vi "MGI Open Window.vi"(8 "error in (no error)":errorcluster, 9 "Center on Caller? (T)":bool=TRUE, 10 "VI To Center On (Caller)":refnum<vi>, 11 "Behavior (Modal)":T1(ring)=enum."Modal") -> (0 "error out":errorcluster, 3 "Open Initially?":bool)   [LabVIEW 2016]
doc: "Sets the caller VI's behavior as specified (modal as default) and opens its front panel. (Useful so you can keep the VI as non-modal most of the time and thus you will not have problems getting stuck with it open).\n\nBy default, centers the opened VI in it's caller VI (if it's open) but that can be changed using the VI To Center On and Center on Caller? inputs.\n\nAuthor: Hope Harrison\nsupport@mooregoodideas.com\nwww.mooregoodideas.com\n\nCopyright (c) 2016, Moore Good Ideas, Inc.\n\nAll rights reserved.\n\nRedistribution and use in source and binary forms, with or without modification, are permitted provided that the following conditions are met:\n\n * Redistributions of source code must retain the above copyright notice, this list of conditions and the following disclaimer.\n * Redistributions in binary form must reproduce the above copyright notice, this list of conditions and the following disclaimer in the documentation and/or other materials provided with the distribution.\n * Neither the name of Moore Good Ideas, Inc. nor the names of its contributors may be used to endorse or promote products derived from this software without specific prior written permission.\n\nTHIS SOFTWARE IS PROVIDED BY THE COPYRIGHT HOLDERS AND CONTRIBUTORS \"AS IS\" AND ANY EXPRESS OR IMPLIED WARRANTIES, INCLUDING, BUT NOT LIMITED TO, THE IMPLIED WARRANTIES OF MERCHANTABILITY AND FITNESS FOR A PARTICULAR PURPOSE ARE DISCLAIMED. IN NO EVENT SHALL THE COPYRIGHT OWNER OR CONTRIBUTORS BE LIABLE FOR ANY DIRECT, INDIRECT, INCIDENTAL, SPECIAL, EXEMPLARY, OR CONSEQUENTIAL DAMAGES (INCLUDING, BUT NOT LIMITED TO, PROCUREMENT OF SUBSTITUTE GOODS OR SERVICES; LOSS OF USE, DATA, OR PROFITS; OR BUSINESS INTERRUPTION) HOWEVER CAUSED AND ON ANY THEORY OF LIABILITY, WHETHER IN CONTRACT, STRICT LIABILITY, OR TORT (INCLUDING NEGLIGENCE OR OTHERWISE) ARISING IN ANY WAY OUT OF THE USE OF THIS SOFTWARE, EVEN IF ADVISED OF THE POSSIBILITY OF SUCH DAMAGE."
uses:
  <userlib>/_MGI/Application Control/MGI VI Reference/MGI Caller's VI Reference.vi
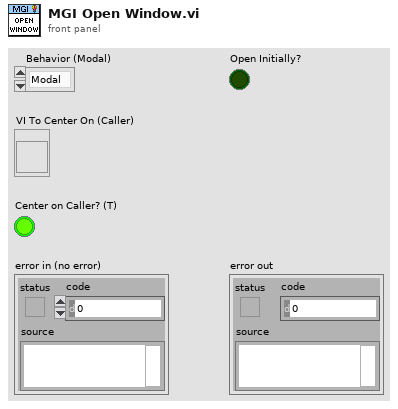
[diagram p1: front panel]
types:
  T1 = enum32{"Invalid", "Default", "Floating", "Floating/Auto-Hide", "Modal"}
  T2 = enum32{"Invalid", "Standard", "Closed", "Hidden", "Minimized", "Maximized"}
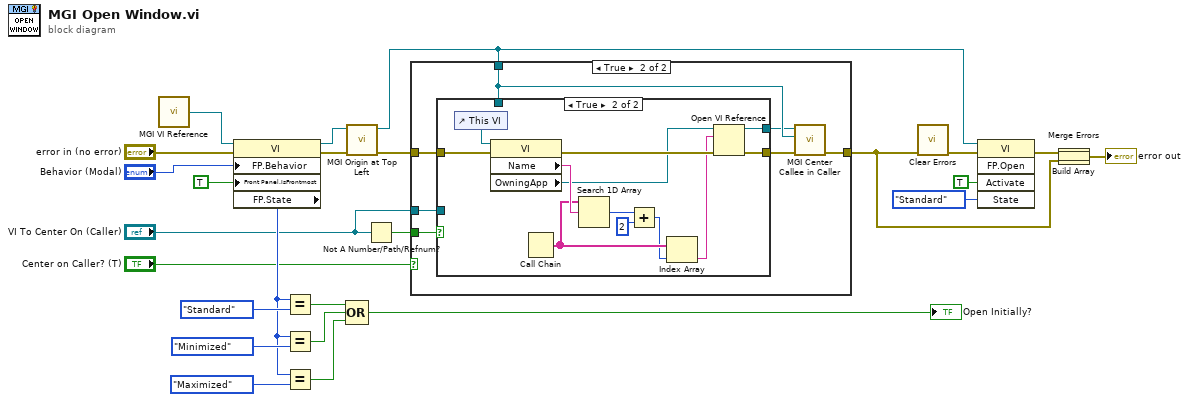
[diagram p0: block diagram]
diagram:
  n1 = call-poly <userlib>:"MGI VI Reference.vi"() -> ("Caller's VI Reference"=w5:refnum<vi>)  [unwired: 1 in]
  n2 = property class="VI"(reference=w5, error in="error in (no error)", "FP.Behavior"="Behavior (Modal)", "Front Panel.IsFrontmost"=TRUE ("Front Panel Window:Is Frontmost")) -> (reference out=w1:refnum<vi>, error out=w4:errorcluster, "FP.State"=w19:T2)
  n3 = Equal?(x=w19, y=T2."Standard" ("Front Panel Window:State")) -> (x = y?=w18:bool)
  n4 = Equal?(x=w19, y=T2."Minimized" ("Front Panel Window:State")) -> (x = y?=w17:bool)
  n5 = Equal?(x=w19, y=T2."Maximized" ("Front Panel Window:State")) -> (x = y?=w16:bool)
  n6 = Compound Arithmetic op=OR(w18, w17, w16) -> (→"Open Initially?":bool)
  n7 = call <userlib>:"MGI Origin at Top Left.vi"("Error In"=w4, "VI Reference In (Caller)"=w1) -> ("Error Out"=w3:errorcluster, "VI Reference Out"=w2:refnum<vi>)  [unwired: 7 in]
  n8 = Not A Number/Path/Refnum?(number/path/refnum="VI To Center On (Caller)") -> (NaN/Path/Refnum?=w9:bool)
  n9 = case shown="True" "Center on Caller? (T)" {
    tunnel: [w27 w30] -> w11
    tunnel: w9 -> [_ w33]
    tunnel: "VI To Center On (Caller)" -> [_ w32]
    tunnel: w2 -> [_ w31]
    tunnel: w3 -> [w27 w34]
    frame False {
    }
    frame True {
      n10 = case shown="True" w33 {
        tunnel: [w35 w42] -> w28
        tunnel: w34 -> [w35 w41]
        tunnel: [w36 w40] -> w29
        tunnel: w32 -> [w36 _]
        tunnel: w31 -> [_ _]
        frame False {
        }
        frame True {
          n11 = control-ref of="This VI"() -> (w37:refnum<vi>)
          n12 = property class="VI"(reference=w37, error in=w41) -> (error out=w47:errorcluster, "Name"=w48:string, "OwningApp"=w44:refnum<vi>)  [unwired: 1 out]
          n13 = Call Chain() -> (call chain=w46:string[])
          n14 = Search 1D Array(1D array=w46, element=w48) -> (index of element=w39:i32)  [unwired: 1 in]
          n15 = Add(x=w39, y=2) -> (x+y=w43:i32)
          n16 = Index Array(array=w46, index=w43) -> (element=w45:string)
          n17 = Open VI Reference(application reference (local)=w44, vi path=w45, error in (no error)=w47) -> (vi reference=w40:refnum<vi>, error out=w42:errorcluster)  [unwired: 3 in]
        }
      }
      n18 = call <userlib>:"MGI Center Callee in Caller.vi"("Error In"=w28, "Callee VI Refnum (Caller)"=w31, "Caller VI Refnum (Callee's Caller)"=w29) -> ("Error Out"=w30:errorcluster)  [unwired: 8 in]
    }
  }
  n19 = call <vilib>:"Clear Errors.vi"("error in (no error)"=w11) -> ("error out"=w13:errorcluster)  [unwired: 5 in, 1 out]
  n20 = invoke class="VI" method="FP.Open"(reference=w2, error in=w13, "Activate"=TRUE ("Activate?"), "State"=T2."Standard") -> (error out=w26:errorcluster)  [unwired: 1 in, 4 out]
  n21 = Build Array(w26, w11) -> (w6:errorcluster[])
  n22 = Merge Errors(w6) -> (→"error out":errorcluster)
